vi "Create Error Injection Test SMO.vi"(7 "Shared Resource (F)":bool, 8 "error in (no error)":errorcluster, 9 "Subsystem Name (optional)":string, 10 "Error code (empty: default)":errorcluster[](array[cluster]), 11 "Inject Errors":T1[](array[typedef])) -> (0 "error out":errorcluster, 1 "SMO name":string, 3 "SMO.ErrorInjection out":refnum<class "SMO.ErrorInjection.lvclass">)   [LabVIEW 2013, in "SMO.ErrorInjection.lvclass"]
uses:
  SMO.ErrorInjection.lvclass
  callback -- enum.ctl
  SMO.ErrorInjection.lvclass/SMO.ErrorInjection.ctl
  src/SMO/SMO.lvclass
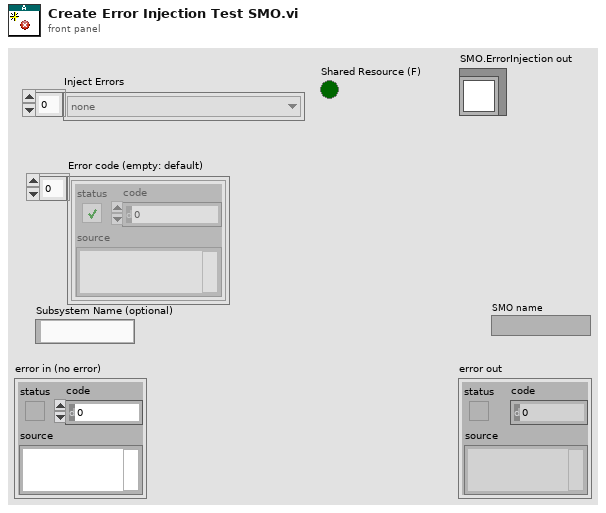
[diagram p1: front panel]
types:
  T1 = typedef "SMO.ErrorInjection.lvclass/callback -- enum.ctl" = enum16{"none", "onCreate", "onCreated", "onStart", "onStarted", "onStop", "onStopped", "onDestroy", "onDestroyed", "Handle Error", "onUnhandledDependencyError", "onDependencyMessage", "onDependencyStarted", "onDependencyStopped", "onOwnershipChanged", "enumerateStaticDependencies", "onProcessStart", "onProcessStarted", "onProcessStartedWithErrors", "onProcessStop", "onProcessStopped", "onProcessKill", "onProcessKilled"}
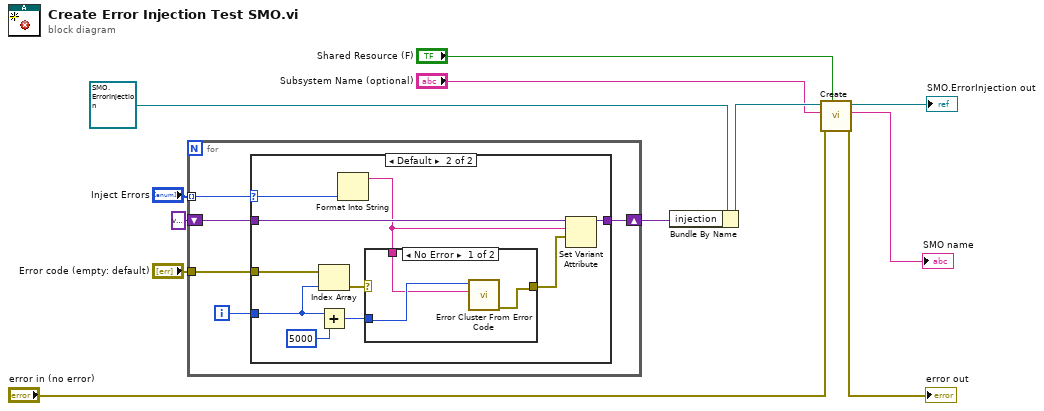
[diagram p0: block diagram]
diagram:
  n1 = for {
    tunnel: "Inject Errors" -> [w13] mode=indexing
    shift-right: [w16] -> w10
    shift-left: variant -> [w17]
    tunnel: "Error code (empty: default)" -> [w15]
    i -> [w14]
    n2 = case shown="Default" w13 {
      selector: w13 -> [_ w19]
      tunnel: w17 -> [w18 w28]
      tunnel: [w18 w27] -> w16
      tunnel: w15 -> [_ w26]
      tunnel: w14 -> [_ w23]
      frame "none" {
      }
      frame Default {
        n3 = Index Array(array=w26, index=w23) -> (element=w25:errorcluster)
        n4 = Add(x=w23, y=5000) -> (x+y=w21:i32)
        n5 = Format Into String(w19) -> (resulting string=w20:string)  [unwired: 3 in, 1 out]
        n6 = case shown="No Error" w25 {
          selector: w25 -> [_ w32]
          tunnel: [w31 w32] -> w24
          tunnel: w21 -> [w30 _]
          tunnel: w20 -> [w29 _]
          frame No Error {
            n7 = call <vilib>:"Error Cluster From Error Code.vi"("error message (\"\")"=w29, "error code (0)"=w30) -> ("error out"=w31:errorcluster)  [unwired: 7 in]
          }
          frame Error {
          }
        }
        n8 = Set Variant Attribute(Variant=w28, name=w20, value=w24) -> (Variant out=w27:variant)  [unwired: 1 in, 2 out]
      }
    }
  }
  n9 = Bundle By Name(cluster=refnum<class "SMO.ErrorInjection.lvclass"> refnum ("SMO.ErrorInjection.lvclass"), "injection"=w10) -> (w5:refnum<class "SMO.ErrorInjection.lvclass">)
  n10 = call "Create.vi"("Shared Resource (F)"="Shared Resource (F)", "error in (no error)"="error in (no error)", "Subsystem Name (optional)"="Subsystem Name (optional)", "SMO"=w5) -> ("error out"=→"error out":errorcluster, "SMO name"=→"SMO name":string, "SMO out"=→"SMO.ErrorInjection out":refnum<class "SMO.ErrorInjection.lvclass">)  [unwired: 5 in]
